vi "init.vi"(8 "error in (no error)":errorcluster, 10 "Scan Settings":T1={"Force Setpoint"=0.0, "Center Point"=413685.4733709468, "Amplitude Scan Settings"={"Start Value"=1.0, "Stop Value"=1.0, "Steps"=2}, "Rate Scan Settings"=[], "Sample Rate"=0.0, "Iterations"=0.0, "Amplitude"=0.0, "Offset"=0.0, "Frequency"=0.0, "Waveform"=enum."Sine Wave", "F1"=0.0, "F2"=0.0, "Duty Cycle"=0.0} {"Amplitude Scan Settings"."Stop Value" format="%.3f"; "Amplitude Scan Settings"."Start Value" format="%.3f"; "Center Point" format="%.3f"; "Force Setpoint" format="%.3f"}, 11 "IWaveformFactory in":refnum<class "IWaveformFactory.lvclass">) -> (0 "error out":errorcluster, 3 "IWaveformFactory out":refnum<class "IWaveformFactory.lvclass">)   [LabVIEW 2015, in "IWaveformFactory.lvclass"]
uses:
  IWaveformFactory.lvclass
  Typedefs/Scan Settings.ctl
  Typedefs/Test Values.ctl
  <userlib>/Common/ILC/Configuration/Scan Rates.ctl
  Typedefs/Waveform.ctl
  Typedefs/FAMTTypedefs.lvlib
  <userlib>/Common/ILC/Configuration/ILCConfiguration.lvlib
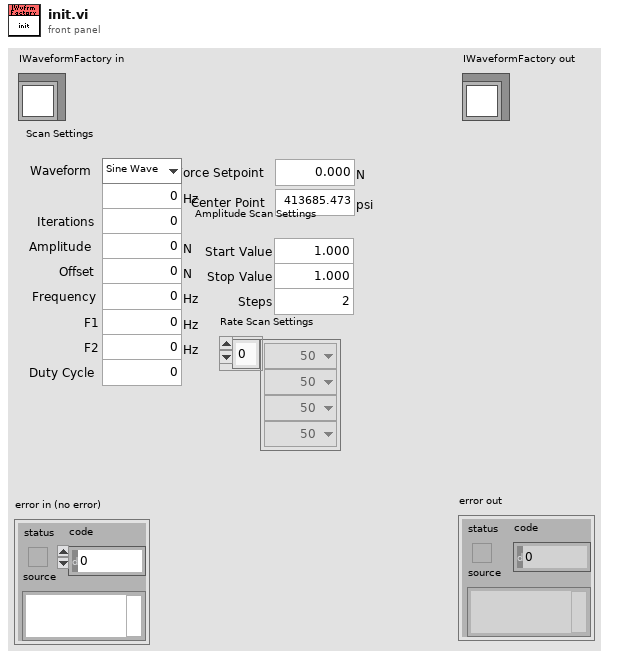
[diagram p1: front panel]
types:
  T1 = typedef "FAMTTypedefs.lvlib/Scan Settings.ctl" = cluster{"Force Setpoint":dbl[unit], "Center Point":dbl[unit], "Amplitude Scan Settings":T2, "Rate Scan Settings":T3[], "Sample Rate":dbl[unit], "Iterations":dbl, "Amplitude":dbl[unit], "Offset":dbl[unit], "Frequency":dbl[unit], "Waveform":T4, "F1":dbl[unit], "F2":dbl[unit], "Duty Cycle":dbl}
  T2 = typedef "FAMTTypedefs.lvlib/Test Values.ctl" = cluster{"Start Value":dbl, "Stop Value":dbl, "Steps":u16}
  T3 = typedef "ILCCommon.lvlib/ILCConfiguration.lvlib/Scan Rates.ctl" = enum16{"50", "60", "100", "120", "200", "240", "300", "400", "480", "600", "1200", "2400", "4800"}
  T4 = typedef "FAMTTypedefs.lvlib/Waveform.ctl" = enum16{"Sine Wave", "Triangle Wave", "Square Wave", "Sawtooth Wave", "Chirp Wave", "Gaussian Wave"}
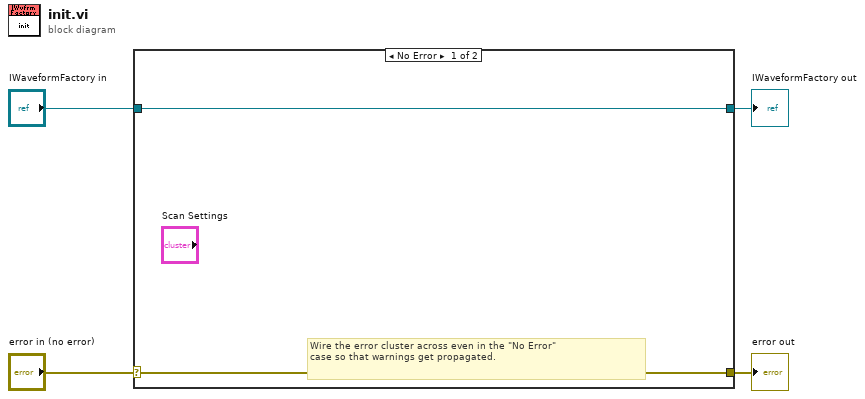
[diagram p0: block diagram]
diagram:
  n1 = case shown="No Error" "error in (no error)" {
    selector: "error in (no error)" -> [w5 w8]
    tunnel: [w5 w8] -> w3
    tunnel: [w6 w7] -> w1
    tunnel: "IWaveformFactory in" -> [w6 w7]
    frame No Error {
      # "Wire the error cluster across even in the \"No Error\"\ncase so that warnings get propagated."
    }
    frame Error {
    }
  }
  "error out" <- w3
  "IWaveformFactory out" <- w1
